vi "LSA.vi"   [LabVIEW 2018]
uses:
  wlmData.dll
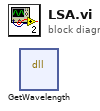
[diagram p0: block diagram]
diagram:
  n1 = dll-call lib="wlmData.dll" fn="GetWavelength"() -> ()  [unwired: 8 in, 2 out]
